vi "Initialize User Event.vi"(8 "error in (no error)":errorcluster, 11 "QControlWizard in":refnum<class "QControl Creation Wizard.lvclass">) -> (0 "error out":errorcluster, 3 "QControlWizard out":refnum<class "QControl Creation Wizard.lvclass">)   [LabVIEW 2015, in "QControl Creation Wizard.lvclass"]
doc: "<b> </b> <b> </b>\n©2016 Q Software Innovations, LLC (QSI)\nwritten by Quentin Alldredge\nproduced in LabVIEW 2015\n\nsupport@qsoftwareinnovations.com\nwww.qsoftwareinnovations.com\n\nAll rights reserved.\n\nRedistribution and use in source and binary forms, with or without modification, are permitted provided that the following conditions are met:\n\n * Redistributions of source code must retain the above copyright notice, this list of conditions and the following disclaimer.\n * Redistributions in binary form must reproduce the above copyright notice, this list of conditions and the following disclaimer in the documentation and/or other materials provided with the distribution.\n * Neither the name of Q Software Innovations, LLC. nor the names of its contributors may be used to endorse or promote products derived from this software without specific prior written permission.\n\nTHIS SOFTWARE IS PROVIDED BY THE COPYRIGHT HOLDERS AND CONTRIBUTORS \"AS IS\" AND ANY EXPRESS OR IMPLIED WARRANTIES, INCLUDING, BUT NOT LIMITED TO, THE IMPLIED WARRANTIES OF MERCHANTABILITY AND FITNESS FOR A PARTICULAR PURPOSE ARE DISCLAIMED. IN NO EVENT SHALL THE COPYRIGHT OWNER OR CONTRIBUTORS BE LIABLE FOR ANY DIRECT, INDIRECT, INCIDENTAL, SPECIAL, EXEMPLARY, OR CONSEQUENTIAL DAMAGES (INCLUDING, BUT NOT LIMITED TO, PROCUREMENT OF SUBSTITUTE GOODS OR SERVICES; LOSS OF USE, DATA, OR PROFITS; OR BUSINESS INTERRUPTION) HOWEVER CAUSED AND ON ANY THEORY OF LIABILITY, WHETHER IN CONTRACT, STRICT LIABILITY, OR TORT (INCLUDING NEGLIGENCE OR OTHERWISE) ARISING IN ANY WAY OUT OF THE USE OF THIS SOFTWARE, EVEN IF ADVISED OF THE POSSIBILITY OF SUCH DAMAGE."
uses:
  QControl Creation Wizard.lvclass
  QControl Creation Wizard.lvclass/QControl Creation Wizard.ctl
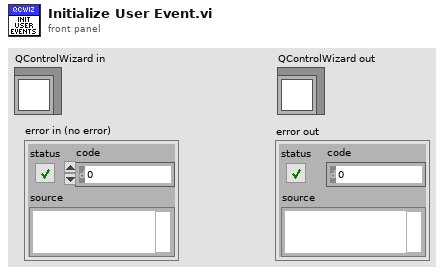
[diagram p1: front panel]
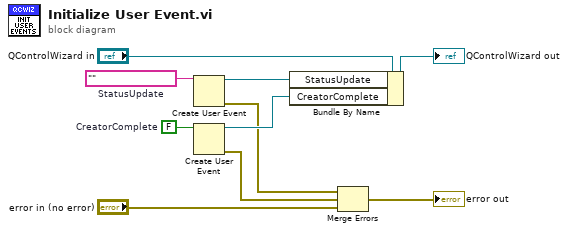
[diagram p0: block diagram]
diagram:
  w4 = FALSE  # CreatorComplete
  w5 = ""  # StatusUpdate
  n1 = Create User Event(user event datatype=w5) -> (user event=w6:refnum<user-event>, error out=w3:errorcluster)  [unwired: 1 in]
  n2 = Create User Event(user event datatype=w4) -> (user event=w9:refnum<user-event>, error out=w2:errorcluster)  [unwired: 1 in]
  n3 = Bundle By Name(cluster="QControlWizard in", "StatusUpdate"=w6, "CreatorComplete"=w9) -> (→"QControlWizard out":refnum<class "QControl Creation Wizard.lvclass">)
  n4 = Merge Errors(w3, w2, "error in (no error)") -> (→"error out":errorcluster)
